vi "Finish.vi"   [LabVIEW 2018]
doc: "This VI is called just before exiting. It is expected to close I/O refnum, save collected data, etc."
uses:
  <vilib>/Rock Robotics/WPI/Utilities/WPI_GetSetVariantRefNum.vi
types:
  T1 = typedef "WPI_MotorControlDeviceRef.ctl" = cluster{"DeviceStatus":errorcluster, "Type":T2, "PWM":cluster{"PWM Channel":T3, "DeadBand":T4}, "CAN":cluster{"Device Number":u8, "SetOutput VI Ref":variant, "GetOutput VI Ref":variant, "Enable VI Ref":variant, "Disable VI Ref":variant, "Data":variant}, "Invert":bool, "DIO PWM":cluster{"PWM \"Enable\" Channel":T3, "DIOChannel":T5, "PWM Rate":dbl}}
  T2 = typedef "WPI_MotorControlType.ctl" = enum16{"PWM", "CAN", "DIO PWM"}
  T3 = typedef "FPGA_DIOPWMChannel.ctl" = enum8{"PWM 0", "PWM 1", "PWM 2", "PWM 3", "PWM 4", "PWM 5", "PWM 6", "PWM 7", "PWM 8", "PWM 9", "PWM MXP 0", "PWM MXP 1", "PWM MXP 2", "PWM MXP 3", "PWM MXP 4", "PWM MXP 5", "PWM MXP 6", "PWM MXP 7", "PWM MXP 8", "PWM MXP 9", "Invalid"}
  T4 = typedef "WPI_PWMDeadband.ctl" = cluster{"Name":string, "maxPositivePwm":i32, "minPositivePwm":i32, "centerPwm":i32, "maxNegativePwm":i32, "minNegativePwm":i32, "angularRange":u16}
  T5 = typedef "FPGA_DIOChannel.ctl" = enum8{"DIO 0", "DIO 1", "DIO 2", "DIO 3", "DIO 4", "DIO 5", "DIO 6", "DIO 7", "DIO 8", "DIO 9", "DIO MXP 0", "DIO MXP 1", "DIO MXP 2", "DIO MXP 3", "DIO MXP 4", "DIO MXP 5", "DIO MXP 6", "DIO MXP 7", "DIO MXP 8", "DIO MXP 9", "DIO MXP 10", "DIO MXP 11", "DIO MXP 12", "DIO MXP 13", "DIO MXP 14", "DIO MXP 15", "SPI Port CS1", "SPI Port CS2", "SPI Port CS3", "SPI Port MISO", "SPI Port MOSI", "Invalid"}
  T6 = typedef "WPI_RobotDriveDevRef.ctl" = cluster{"DevStatus":errorcluster, "Motors[]":T1[], "Square Inputs":bool, "Max Output":dbl}
  T7 = typedef "WPI_JoystickDevRef.ctl" = cluster{"Device":T8}
  T8 = typedef "WPI_JoystickDeviceEnum.ctl" = enum16{"USB 0", "USB 1", "USB 2", "USB 3", "USB 4", "USB 5"}
  T9 = typedef "WPI_GyroDevRef.ctl" = cluster{"DevStatus":errorcluster, "Analog Channel":T10, "Gain (VoltsPerDegree/Second)":dbl, "Gyro Type":enum16{"Analog", "XRS450"}, "Handle":i32, "SPI Bus":T11, "Device Found":bool, "Sample Rate":dbl, "Calibrate On Open":bool, "Offset":dbl}
  T10 = typedef "FPGA_AIChannel.ctl" = enum8{"AI 0", "AI 1", "AI 2", "AI 3", "AI MXP 0", "AI MXP 1", "AI MXP 2", "AI MXP 3", "Invalid"}
  T11 = typedef "spi_bus.ctl" = enum16{"SPI On-Board, CS0", "SPI On-Board, CS1", "SPI On-Board, CS2", "SPI On-Board, CS3", "SPI MXP", "Invalid"}
  T12 = typedef "WPI_SolenoidDevRef.ctl" = cluster{"DevStatus":errorcluster, "Pneumatics Control Module":u8, "Forward Solenoid Channel":T13, "Reverse Solenoid Channel":T13}
  T13 = typedef "WPI_SolenoidChannel.ctl" = enum8{"Solenoid 0", "Solenoid 1", "Solenoid 2", "Solenoid 3", "Solenoid 4", "Solenoid 5", "Solenoid 6", "Solenoid 7", "Invalid"}
  T14 = typedef "WPI_CompressorDevRef.ctl" = cluster{"DevStatus":errorcluster, "Pneumatics Control Module":u8}
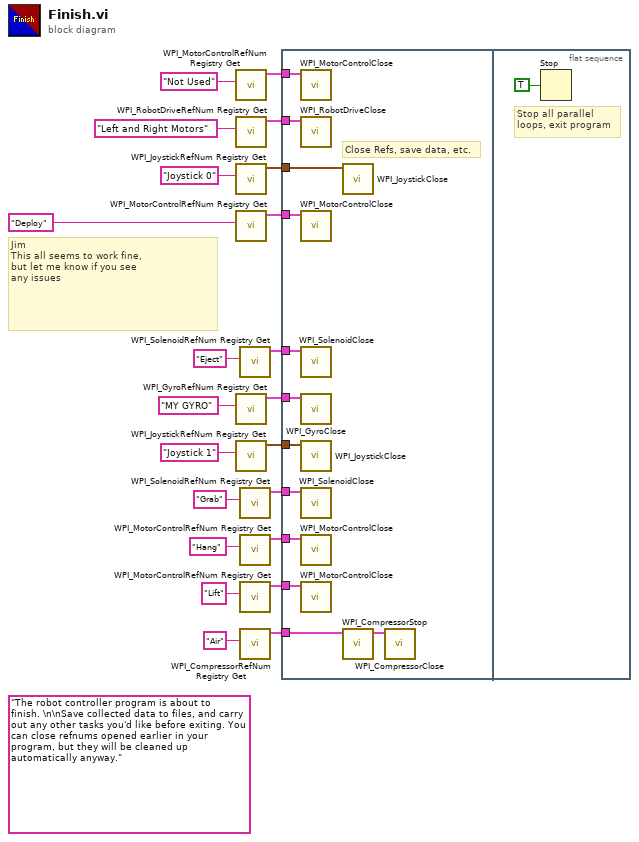
[diagram p0: block diagram]
diagram:
  (unwired) "The robot controller program is about to finish. \n\nSave collected data to files, and carry out any other tasks you'd like before exiting. You can close refnums opened earlier in your program, but they will be cleaned up automatically anyway."
  # "Jim\nThis all seems to work fine,\nbut let me know if you see\nany issues"
  n1 = call <vilib>:"WPI_MotorControlRefNum Registry Get.vi"("refnum name"="Not Used") -> ("MotorControlDevRef"=w10:T1)  [unwired: 9 in, 1 out]
  n2 = call <vilib>:"WPI_RobotDriveRefNum Registry Get.vi"("refnum name"="Left and Right Motors") -> ("RobotDriveDevRef"=w20:T6)  [unwired: 1 in, 9 out]
  n3 = call <vilib>:"WPI_JoystickRefNum Registry Get.vi"("refnum name"="Joystick 0") -> ("JoystickDevRef"=w14:T7)  [unwired: 1 in, 9 out]
  n4 = call <vilib>:"WPI_MotorControlRefNum Registry Get.vi"("refnum name"="Deploy") -> ("MotorControlDevRef"=w15:T1)  [unwired: 9 in, 1 out]
  n5 = call <vilib>:"WPI_GyroRefNum Registry Get.vi"("refnum name"="MY GYRO") -> ("GyroDevRef"=w19:T9)  [unwired: 9 in, 1 out]
  n6 = call <vilib>:"WPI_JoystickRefNum Registry Get.vi"("refnum name"="Joystick 1") -> ("JoystickDevRef"=w13:T7)  [unwired: 1 in, 9 out]
  n7 = call <vilib>:"WPI_SolenoidRefNum Registry Get.vi"("refnum name"="Eject") -> ("SolenoidDevRef"=w3:T12)  [unwired: 9 in, 1 out]
  n8 = call <vilib>:"WPI_SolenoidRefNum Registry Get.vi"("refnum name"="Grab") -> ("SolenoidDevRef"=w4:T12)  [unwired: 9 in, 1 out]
  n9 = call <vilib>:"WPI_MotorControlRefNum Registry Get.vi"("refnum name"="Hang") -> ("MotorControlDevRef"=w9:T1)  [unwired: 9 in, 1 out]
  n10 = call <vilib>:"WPI_MotorControlRefNum Registry Get.vi"("refnum name"="Lift") -> ("MotorControlDevRef"=w12:T1)  [unwired: 9 in, 1 out]
  n11 = call <vilib>:"WPI_CompressorRefNum Registry Get.vi"("refnum name"="Air") -> ("CompressorDevRef"=w5:T14)  [unwired: 9 in, 1 out]
  n12 = flat-sequence {
    tunnel: w20 -> [w34]
    tunnel: w19 -> [w33]
    tunnel: w15 -> [w30]
    tunnel: w14 -> [w32]
    tunnel: w13 -> [w31]
    tunnel: w12 -> [w29]
    tunnel: w10 -> [w28]
    tunnel: w9 -> [w27]
    tunnel: w5 -> [w25]
    tunnel: w4 -> [w24]
    tunnel: w3 -> [w23]
    frame #0 {
      # "Close Refs, save data, etc."
      n13 = call <vilib>:"WPI_MotorControlClose.vi"("MotorControlDevRef"=w28) -> ()  [unwired: 10 in, 1 out]
      n14 = call <vilib>:"WPI_RobotDriveClose.vi"("RobotDriveDevRef"=w34) -> ()  [unwired: 1 in, 10 out]
      n15 = call <vilib>:"WPI_MotorControlClose.vi"("MotorControlDevRef"=w30) -> ()  [unwired: 10 in, 1 out]
      n16 = call <vilib>:"WPI_SolenoidClose.vi"("SolenoidDevRef"=w23) -> ()  [unwired: 10 in, 1 out]
      n17 = call <vilib>:"WPI_GyroClose.vi"("GyroDevRef"=w33) -> ()  [unwired: 10 in, 1 out]
      n18 = call <vilib>:"WPI_JoystickClose.vi"("JoystickDevRef"=w31) -> ()  [unwired: 11 out]
      n19 = call <vilib>:"WPI_SolenoidClose.vi"("SolenoidDevRef"=w24) -> ()  [unwired: 10 in, 1 out]
      n20 = call <vilib>:"WPI_MotorControlClose.vi"("MotorControlDevRef"=w27) -> ()  [unwired: 10 in, 1 out]
      n21 = call <vilib>:"WPI_MotorControlClose.vi"("MotorControlDevRef"=w29) -> ()  [unwired: 10 in, 1 out]
      n22 = call <vilib>:"WPI_JoystickClose.vi"("JoystickDevRef"=w32) -> ()  [unwired: 11 out]
      n23 = call <vilib>:"WPI_CompressorStop.vi"("CompressorDevRef"=w25) -> ("CompressorDevRef"=w26:T14)  [unwired: 9 in, 1 out]
      n24 = call <vilib>:"WPI_CompressorClose.vi"("CompressorDevRef"=w26) -> ()  [unwired: 10 in, 1 out]
    }
    frame #1 {
      # "Stop all parallel\nloops, exit program"
      n25 = Stop(stop? (T)=TRUE ("Quit")) -> ()
    }
  }
